vi "Set Add To Project ComboBox.vi"(8 "Error In":errorcluster, 10 "Project Names":string[](array[string]), 11 "Project Name ComboBox Ref":refnum<vi>) -> (0 "Error Out":errorcluster)   [LabVIEW 2022 SP3]
doc: "<add documentation here>"
uses:
  <vilib>/Utility/miscctls.llb/LVFontTypeDef.ctl
panel:
  # "Development\nControls or indicators that are useful for development or testing, but which are not outputs of the VI."
  # "Input\nInputs to the VI"
  # "Output\nOutputs of the VI"
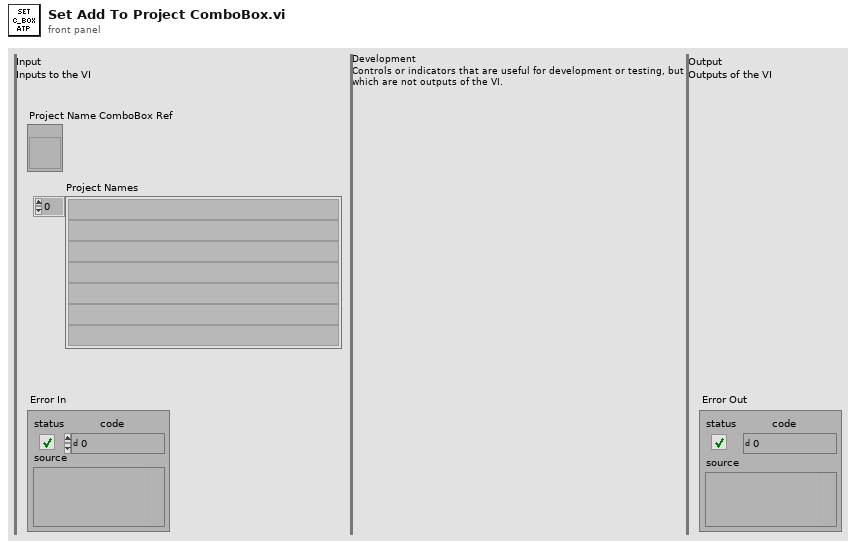
[diagram p1: front panel]
types:
  T1 = typedef "LVFontTypeDef.ctl" = cluster{"Font Name":string, "Size":u16, "Bold":bool, "Italic":bool, "Underline":bool, "Strikeout":bool, "Color":u32}
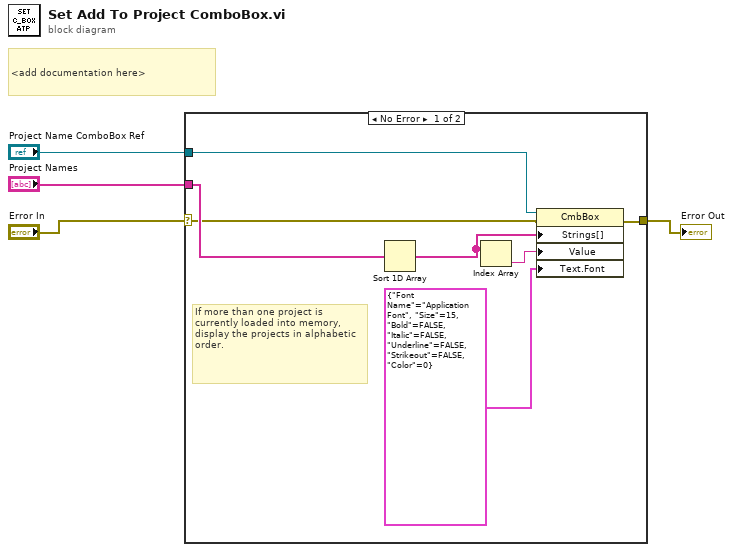
[diagram p0: block diagram]
diagram:
  # "<add documentation here>"
  n1 = case shown="No Error" "Error In" {
    selector: "Error In" -> [w6 w12]
    tunnel: [w5 w12] -> w3
    tunnel: "Project Name ComboBox Ref" -> [w10 _]
    tunnel: "Project Names" -> [w9 _]
    frame No Error {
      # "If more than one project is currently loaded into memory, display the projects in alphabetic order."
      n2 = Sort 1D Array(array=w9) -> (sorted array=w7:string[])
      n3 = Index Array(array=w7) -> (element=w8:string)  [unwired: 1 in]
      n4 = property class="CmbBox"(reference=w10, error in=w6, "Strings[]"=w7, "Value"=w8, "Text.Font"=T1 {"Font Name"="Application Font", "Size"=15, "Bold"=FALSE, "Italic"=FALSE, "Underline"=FALSE, "Strikeout"=FALSE, "Color"=0}) -> (error out=w5:errorcluster)  [unwired: 1 out]
    }
    frame Error {
    }
  }
  "Error Out" <- w3
